vi "RT Loop - Analyze Acceleration.vi"(7 "testing":bool, 8 "error in (no error)":errorcluster, 9 "Acceleration RT FIFO In":T1, 10 "FPGA VI Reference Out":refnum<k20>, 11 "Message Queue":refnum<queue>) -> (1 "Acceleration RT FIFO Out":T1)   [LabVIEW 2017]
doc: "Read and analyze acceleration waveform data from FPGA via DMA FIFO. If the acceleration is over the limit, then send the acceleration waveform data to the Log Data Loop."
uses:
  UI Error Handlers/support/Message Queue/Message Cluster.ctl
  controls/Acceleration RT FIFO Reference.ctl
  Globals/Global - All RT Loop Stop.vi
  Globals/Global - Configuration Options.vi
  <vilib>/Utility/error.llb/Error Cluster From Error Code.vi
  <vilib>/rvi/errors/niLvFpgaAdjustHostInterfaceError.vi
  <vilib>/rvi/interface/nirviMethod/nirviMethod.xnode
  <vilib>/FPGAPlugInAG/Dynamic/niLvFpga_ReadFifo_Dynamic.vi
  <vilib>/rvi/errors/niLvFpgaMergeErrorWithErrorCode.vi
  UI Error Handlers/support/Message Queue/Message Queue.lvlib
panel:
  out "G1 status.G1 trigger 2":bool
  out "G1 status":cluster{"G1 trigger":bool}
  out "G1 status.G1 trigger":bool
  out "sta":bool
  out "logical OR":bool
  in  "Data Rate (Hz)":dbl
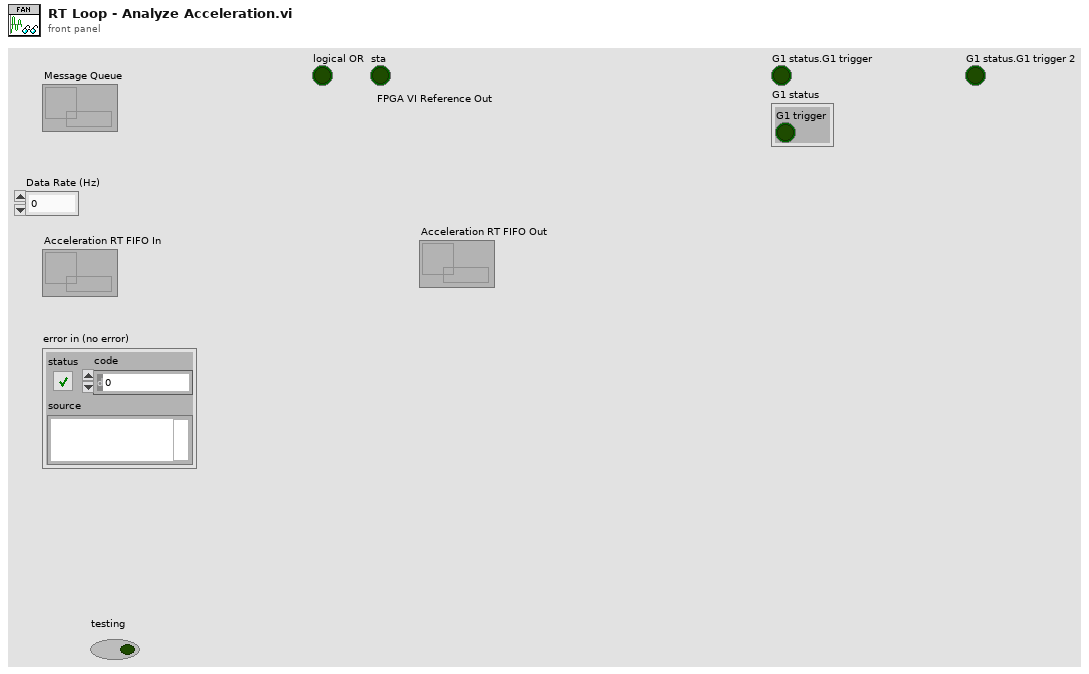
[diagram p1: front panel]
types:
  T1 = typedef "Acceleration RT FIFO Reference.ctl" = refnum<k33>
  T2 = cluster{"Tool data":cluster{"Number of teeth":sgl}, "Cutting data":cluster{"rpm":sgl}, "Limits":cluster{"Magnitude threshold":sgl, "Tolerance":sgl}, "G1 status":cluster{"G1 trigger":bool}}
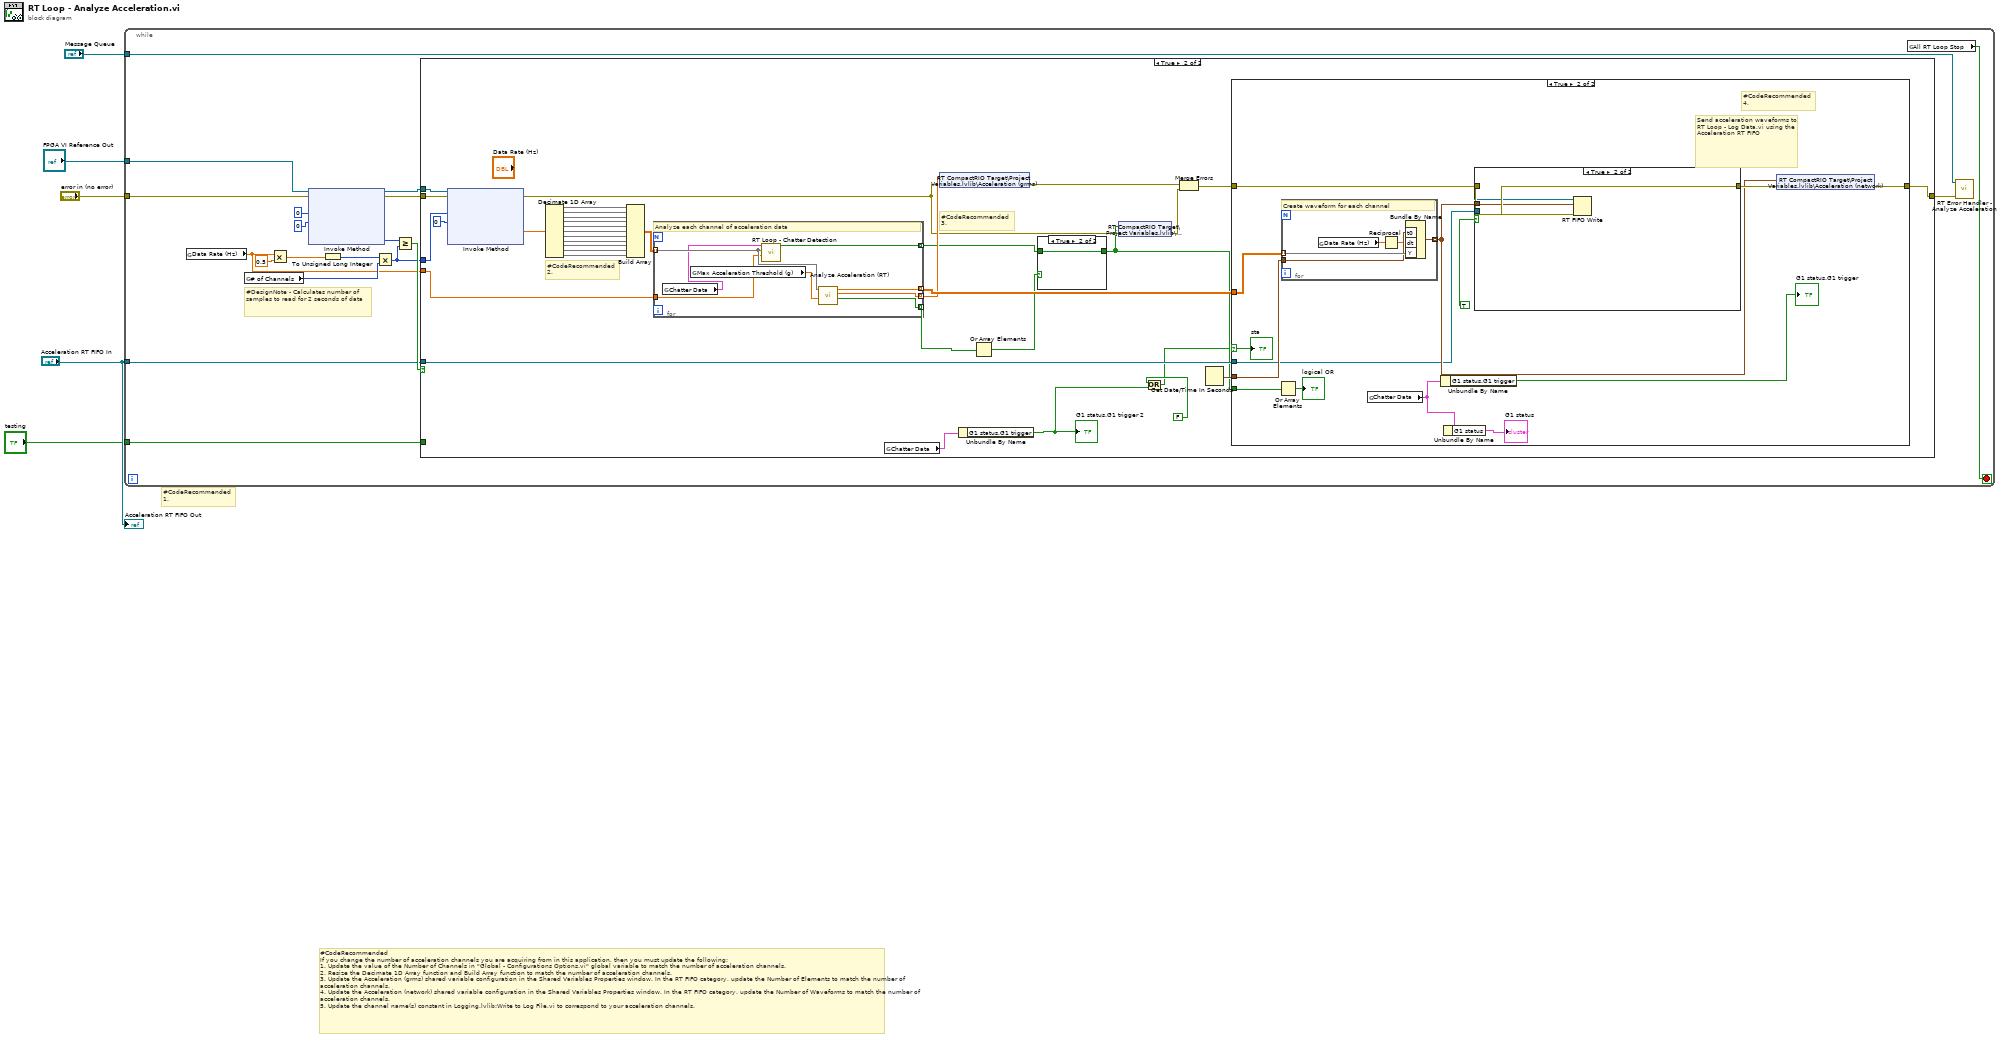
[diagram p0: block diagram]
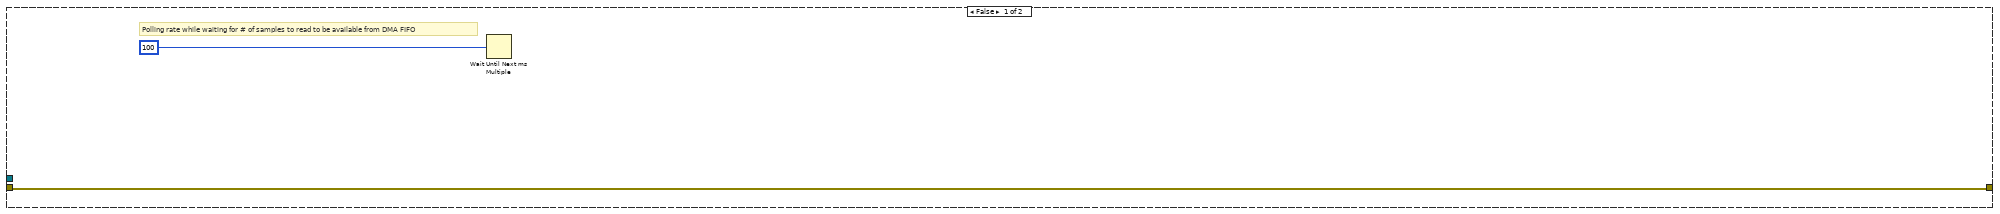
[diagram p2: hidden frame]
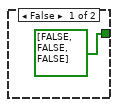
[diagram p3: hidden frame]
diagram:
  # "#CodeRecommended\n1."
  # "#CodeRecommended\nIf you change the number of acceleration channels you are acquiring from in this application, then you must update the following:\n1. Update the value of the Number of Channels in \"Global - Configurations Options.vi\" global variable to match the number of acceleration channels.\n2. Resize the Decimate 1D Array function and Build Array function to match the number of acceleration channels. \n3. Update the Acceleration (grms) shared variable configuration in the Shared Variables Properties window. In the RT FIFO category, update the Number of Elements to match the number of acceleration channels. \n4. Update the Acceleration (network) shared variable configuration in the Shared Variables Properties window. In the RT FIFO category, update the Number of Waveforms to match the number of acceleration channels.\n5. Update the channel name(s) constant in Logging.lvlib:Write to Log File.vi to correspond to your acceleration channels."
  n1 = while {
    tunnel: "FPGA VI Reference Out" -> [w24]
    tunnel: "error in (no error)" -> [w23]
    tunnel: "Message Queue" -> [w16]
    tunnel: "Acceleration RT FIFO In" -> [w14]
    tunnel: "testing" -> [w6]
    stop <- w17 stop-if-true
    # "#DesignNote - Calculates number of samples to read for 2 seconds of data"
    n2 = global read "Global - Configuration Options.vi" "Data Rate (Hz)"() -> (w8:dbl)
    n3 = global read "Global - Configuration Options.vi" "# of Channels"() -> (w9:u32)
    n4 = Multiply(x=w8, y=0.5) -> (x*y=w12:dbl)
    n5 = xnode "Invoke Method"("FPGA VI Reference In"=w24, "error in"=w23, "Number of Elements"=u32 0, "Timeout (ms)"=0) -> ("FPGA VI Reference Out"=w20:refnum<k20>, "error out"=w19:errorcluster, "Elements Remaining"=w7:u32)  [unwired: 1 out]
    n6 = To Unsigned Long Integer(number=w12) -> (unsigned 32bit integer=w11:u32)
    n7 = Multiply(x=w11, y=w9) -> (x*y=w10:u32)
    n8 = Greater Or Equal?(x=w7, y=w10) -> (x >= y?=w18:bool)
    n9 = case shown="True" w18 {
      tunnel: w20 -> [_ w61]
      tunnel: w19 -> [w26 w60]
      tunnel: [w26 w56] -> w15
      tunnel: w10 -> [_ w59]
      tunnel: w14 -> [_ w54]
      tunnel: w8 -> [_ w46]
      tunnel: w6 -> [_ _]
      frame False {
        # "Polling rate while waiting for # of samples to read to be available from DMA FIFO"
        n10 = Wait Until Next ms Multiple(millisecond multiple=u32 100) -> ()  [unwired: 1 out]
      }
      frame True {
        # "#CodeRecommended\n3."
        # "#CodeRecommended\n2."
        n11 = xnode "Invoke Method"("FPGA VI Reference In"=w61, "error in"=w60, "Number of Elements"=w59, "Timeout (ms)"=0) -> ("error out"=w45:errorcluster, "Data"=w53:sgl[])  [unwired: 2 out]
        n12 = Decimate 1D Array(w53) -> (w52:sgl[], w51:sgl[], w48:sgl[], w38:sgl[], w37:sgl[], w36:sgl[], w35:sgl[], w34:sgl[], w33:sgl[], w32:sgl[], w31:sgl[])
        n13 = Build Array(w52, w51, w48, w38, w37, w36, w35, w34, w33, w32, w31) -> (w50:sgl[][])
        n14 = for {
          tunnel: [w71] -> w55 mode=indexing
          tunnel: [w70] -> w49 mode=indexing
          tunnel: [w69] -> w47 mode=indexing
          tunnel: w50 -> [w67] mode=indexing
          tunnel: w46 -> [w66]
          tunnel: [w65] -> w40 mode=indexing
          # "Analyze each channel of acceleration data"
          n15 = global read "Global - Configuration Options.vi" "Chatter Data"() -> (w64:T2)
          n16 = global read "Global - Configuration Options.vi" "Max Acceleration Threshold (g)"() -> (w68:sgl)
          n17 = call "RT Loop - Chatter Detection.vi"("Data Rate (Hz)"=w66, "Acceleration Waveform (SGL)"=w67, "Chatter Data"=w64) -> ("Chatter?"=w65:bool)  [unwired: 8 in]
          n18 = call "Analyze Acceleration (RT).vi"("Max Instantaneous Acceleration (g)"=w68, "Acceleration Waveform (SGL)"=w67) -> ("Over Limit?"=w71:bool, "Acceleration (grms)"=w69:dbl, "Acceleration Waveform (DBL)"=w70:dbl[])  [unwired: 7 in]
        }
        n19 = global read "Global - Configuration Options.vi" "Chatter Data"() -> (w30:T2)
        n20 = shared-variable "RT CompactRIO Target\\Project Variables.lvlib\\Acceleration (grms)"(w47, error in=w45) -> (error out=w43:errorcluster)
        n21 = Unbundle By Name(w30) -> ("G1 status.G1 trigger"=w29:bool)
        "G1 status.G1 trigger 2" <- w29
        n22 = Or Array Elements(Boolean array=w55) -> (logical OR=w41:bool)
        n23 = case shown="True" w41 {
          tunnel: w40 -> [_ w63]
          tunnel: [bool[] [FALSE, FALSE, FALSE] ("Chatter?") w63] -> w39
          frame False {
          }
          frame True {
          }
        }
        n24 = shared-variable "RT CompactRIO Target\\Project Variables.lvlib\\Chatter?"(w39, error in=w45) -> (error out=w44:errorcluster)
        n25 = Or(x=FALSE, y=w29) -> (x .or. y?=w27:bool)
        n26 = Merge Errors(w43, w44) -> (w42:errorcluster)
        n27 = Get Date/Time In Seconds() -> (seconds since 1Jan1904=w57:timestamp)
        n28 = case shown="True" w27 {
          selector: w27 -> [_ w77]
          tunnel: w57 -> [_ w86]
          tunnel: w42 -> [w72 w85]
          tunnel: [w72 w83] -> w56
          tunnel: w54 -> [_ w81]
          tunnel: w49 -> [_ w80]
          tunnel: w39 -> [_ w78]
          frame False {
          }
          frame True {
            # "#CodeRecommended\n4."
            # "Send acceleration waveforms to RT Loop - Log Data.vi using the Acceleration RT FIFO"
            n29 = Or Array Elements(Boolean array=w78) -> (logical OR=→"logical OR":bool)
            n30 = for {
              tunnel: w80 -> [w96] mode=indexing
              tunnel: w86 -> [w95]
              tunnel: [w93] -> w82 mode=indexing
              # "Create waveform for each channel"
              n31 = global read "Global - Configuration Options.vi" "Data Rate (Hz)"() -> (w92:dbl)
              n32 = Reciprocal(x=w92) -> (1/x=w94:dbl)
              n33 = Bundle By Name("t0"=w95, "dt"=w94, "Y"=w96) -> (w93:waveform(dbl))  [unwired: 1 in]
            }
            n34 = global read "Global - Configuration Options.vi" "Chatter Data"() -> (w76:T2)
            n35 = Unbundle By Name(w76) -> ("G1 status.G1 trigger"=→"G1 status.G1 trigger":bool)
            n36 = Unbundle By Name(w76) -> ("G1 status"=→"G1 status":cluster{"G1 trigger":bool})
            n37 = case shown="True" TRUE {
              tunnel: w85 -> [w87 w91]
              tunnel: [w87 w90] -> w84
              tunnel: w82 -> [_ w89]
              tunnel: w81 -> [_ w88]
              frame False {
              }
              frame True {
                n38 = RT FIFO Write(0:w88, 1:w89, 3:w91) -> (11:w90:errorcluster)  [unwired: 2 in, 3 out]
              }
            }
            n39 = shared-variable "RT CompactRIO Target\\Project Variables.lvlib\\Acceleration (network)"(w82, error in=w84) -> (error out=w83:errorcluster)
            "sta" <- w77
          }
        }
      }
    }
    n40 = global read "Global - All RT Loop Stop.vi" "All RT Loop Stop"() -> (w17:bool)
    n41 = call "RT Error Handler - Analyze Acceleration.vi"("error in (no error)"=w15, "Message Queue"=w16) -> ()  [unwired: 9 in, 1 out]
  }
  "Acceleration RT FIFO Out" <- "Acceleration RT FIFO In"
